vi "SaveMeasure.vi"(6 "EN":bool, 8 "Space":T1, 9 "Measure":T2, 10 "Measure Name":string(combo)="DL", 11 "MasterPath":path=path "D:/Output") -> (0 "SaveOK":bool, 1 "File path":path, 3 "Folder path":path)   [LabVIEW 2017]
uses:
  <vilib>/Utility/file.llb/Write Delimited Spreadsheet (string).vi
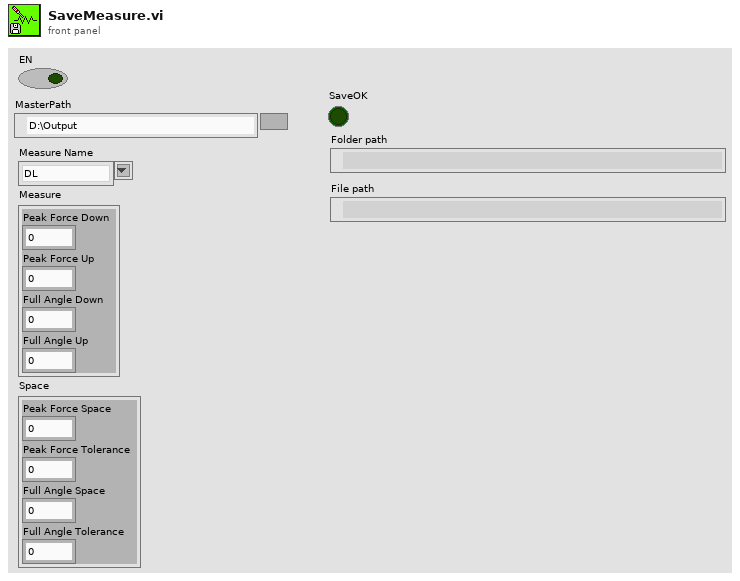
[diagram p1: front panel]
types:
  T1 = cluster{"Peak Force Space":dbl, "Peak Force Tolerance":dbl, "Full Angle Space":dbl, "Full Angle Tolerance":dbl}
  T2 = cluster{"Peak Force Down":dbl, "Peak Force Up":dbl, "Full Angle Down":dbl, "Full Angle Up":dbl}
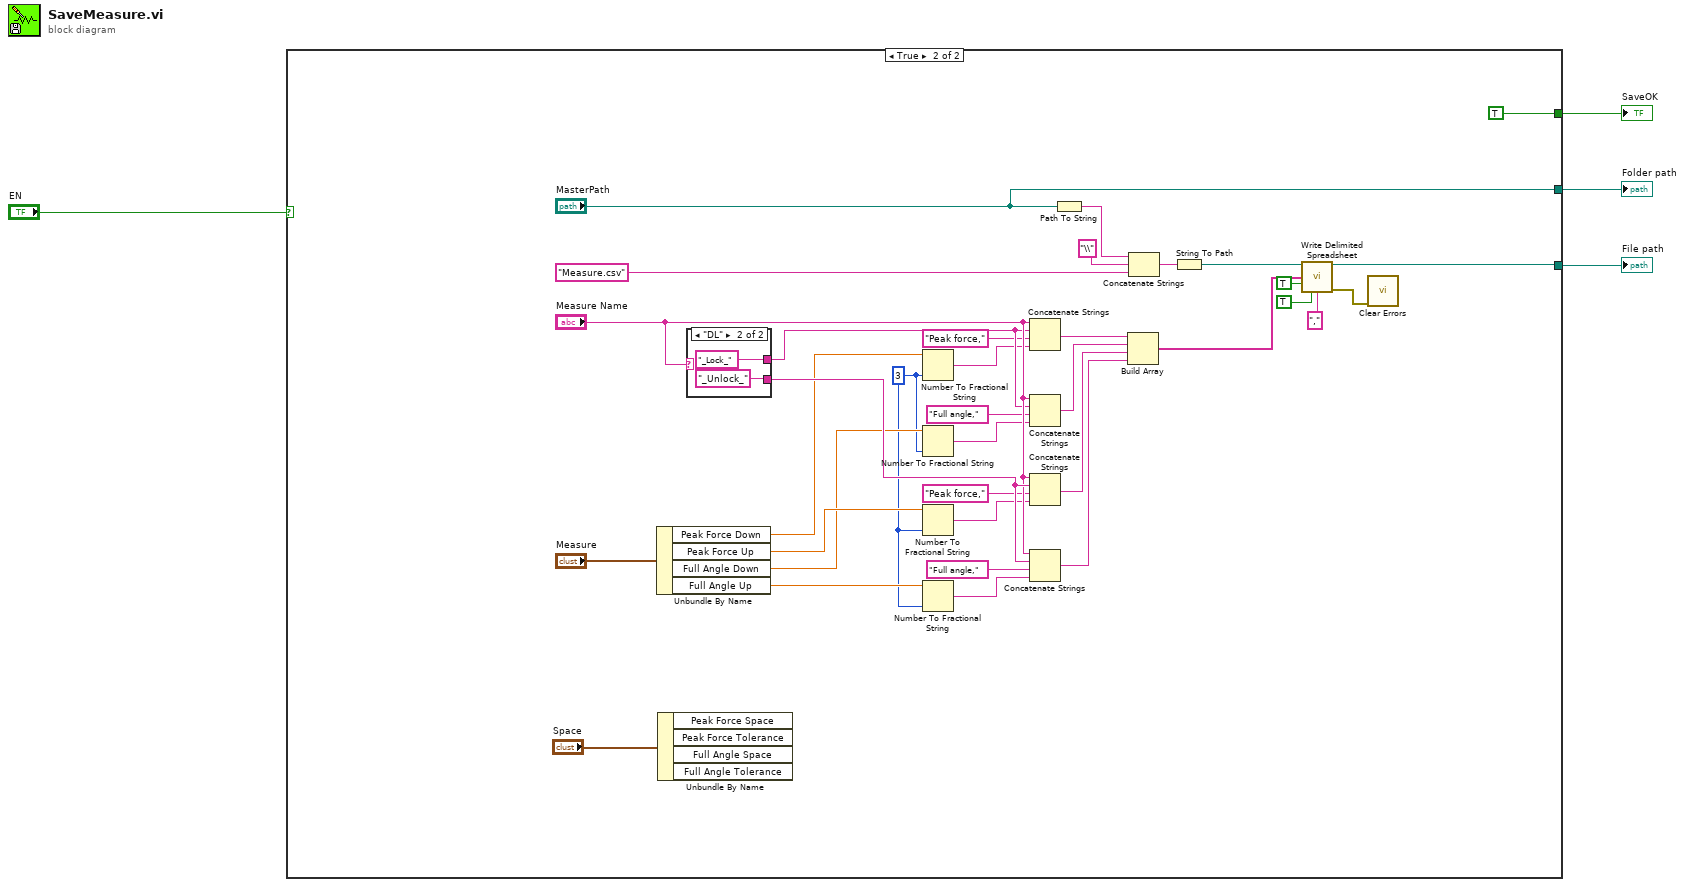
[diagram p0: block diagram]
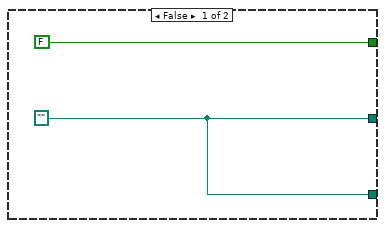
[diagram p2: hidden frame]
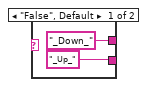
[diagram p3: hidden frame]
diagram:
  n1 = case shown="True" "EN" {
    tunnel: [w5 "MasterPath"] -> w4
    tunnel: [FALSE TRUE] -> w3
    tunnel: [w5 w39] -> w2
    frame False {
      w5 = path ""
    }
    frame True {
      w13 = i16 3 ("precision (6)")
      n2 = Unbundle By Name("Measure") -> ("Peak Force Down"=w15:dbl, "Peak Force Up"=w28:dbl, "Full Angle Down"=w20:dbl, "Full Angle Up"=w29:dbl)
      n3 = Unbundle By Name("Space") -> ()  [unwired: 4 out]
      n4 = case shown="\"DL\"" "Measure Name" {
        tunnel: ["_Down_" ("string") "_Lock_" ("string")] -> w19
        tunnel: ["_Up_" ("string") "_Unlock_" ("string")] -> w25
        frame "False", Default {
        }
        frame "DL" {
        }
      }
      n5 = Number To Fractional String(number=w15, precision (6)=w13) -> (F-format string=w16:string)  [unwired: 2 in]
      n6 = Number To Fractional String(number=w20, precision (6)=w13) -> (F-format string=w18:string)  [unwired: 2 in]
      n7 = Number To Fractional String(number=w28, precision (6)=w13) -> (F-format string=w23:string)  [unwired: 2 in]
      n8 = Number To Fractional String(number=w29, precision (6)=w13) -> (F-format string=w22:string)  [unwired: 2 in]
      n9 = Concatenate Strings("Measure Name", w19, "Peak force," ("string"), w16) -> (w17:string)
      n10 = Concatenate Strings("Measure Name", w19, "Full angle," ("string"), w18) -> (w21:string)
      n11 = Concatenate Strings("Measure Name", w25, "Peak force," ("string"), w23) -> (w26:string)
      n12 = Concatenate Strings("Measure Name", w25, "Full angle," ("string"), w22) -> (w27:string)
      n13 = Path To String(path="MasterPath") -> (string=w30:string)
      n14 = Build Array(w17, w21, w26, w27) -> (w8:string[])
      n15 = Concatenate Strings(w30, "\\" ("string"), "Measure.csv" ("string")) -> (w35:string)
      n16 = String To Path(string=w35) -> (path=w34:path)
      n17 = call-poly <vilib>:"Write Delimited Spreadsheet.vi"("file path (dialog if empty)"=w34, "1D data"=w8, "append to file? (new file:F)"=TRUE, "transpose? (no:F)"=TRUE, "delimiter (\\t)"="," ("delimiter (\\t)")) -> ("new file path (Not A Path if cancelled)"=w39:path, "error out"=w32:errorcluster)  [unwired: 9 in]
      n18 = call <vilib>:"Clear Errors.vi"("error in (no error)"=w32) -> ()  [unwired: 5 in, 2 out]
    }
  }
  "Folder path" <- w4
  "SaveOK" <- w3
  "File path" <- w2
